vi "Generate Reflection Matrix.vi"(1 "Bit":bool) -> (0 "Reflection Matrix":T1)   [LabVIEW 2019, in "Referential.lvclass"]
uses:
  Referential.lvclass
  <vilib>/Analysis/Matrix/Datatypes/RealMatrix.ctl
  <vilib>/Analysis/Matrix/NI_Matrix.lvlib
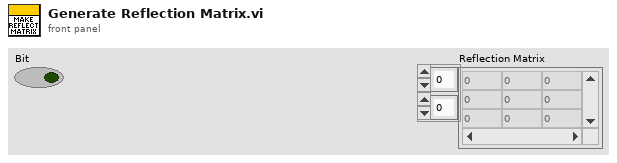
[diagram p1: front panel]
types:
  T1 = typedef "NI_Matrix.lvlib/RealMatrix.ctl" = dbl[][]
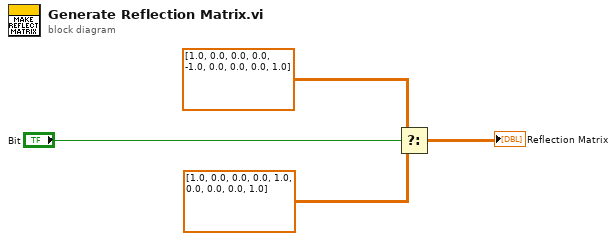
[diagram p0: block diagram]
diagram:
  n1 = Select(t=T1 [[1.0, 0.0, 0.0], [0.0, -1.0, 0.0], [0.0, 0.0, 1.0]] ("appended array"), s="Bit", f=T1 [[1.0, 0.0, 0.0], [0.0, 1.0, 0.0], [0.0, 0.0, 1.0]] ("appended array")) -> (s? t:f=→"Reflection Matrix":T1)
